vi "Set Message2 Text Html.vi"(0 "handles cluster in":T1 caption="ハンドルクラスター入力", 5 "subject":string caption="件名", 7 "plain text message":string caption="標準テキストメッセージ", 9 "html message":string caption="htmlメッセージ", 11 "error in (no error)":errorcluster caption="エラー入力（エラーなし）") -> (4 "handles cluster out":T1 caption="ハンドルクラスター出力", 15 "error out":errorcluster caption="エラー出力")   [LabVIEW 2015]
doc: "Eメールの本文に含めるテキストとHTMLを設定します。\nメールは「multipart」となり、標準テキストメッセージが「content-type: text/plain」に、htmlメッセージが「content-type: text/html」となる。"
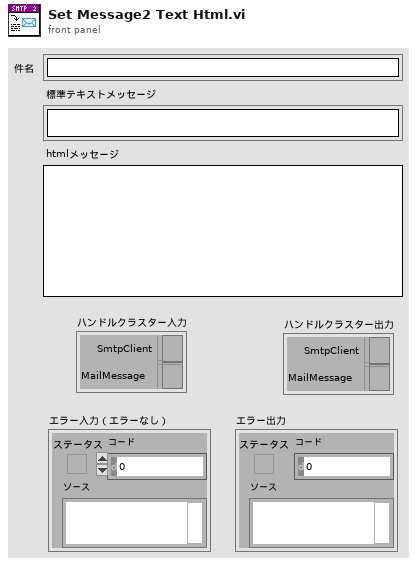
[diagram p1: front panel]
types:
  T1 = cluster{"SmtpClient":refnum<k24>, "MailMessage":refnum<k24>}
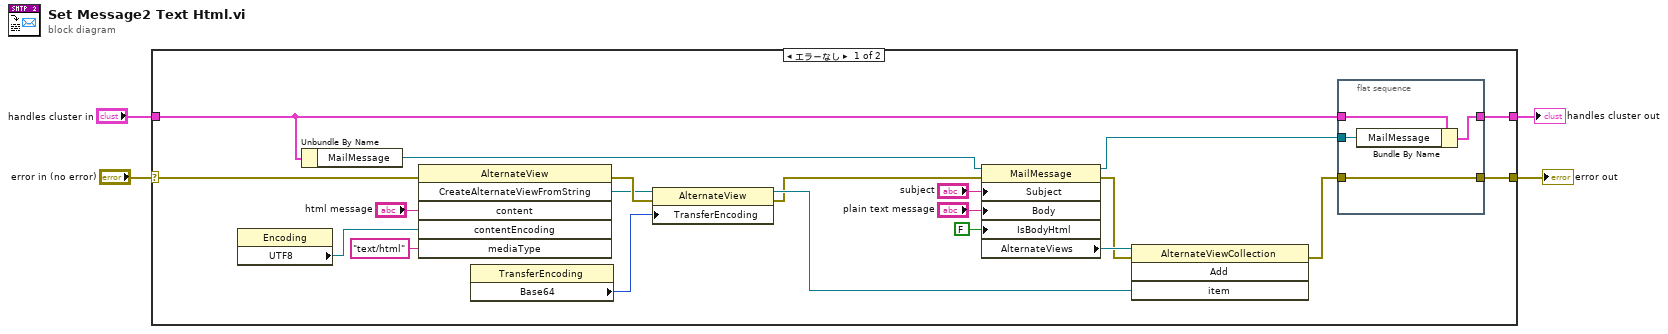
[diagram p0: block diagram]
diagram:
  n1 = case shown="エラーなし" "error in (no error)" {
    selector: "error in (no error)" -> [w16 w30]
    tunnel: [w12 w30] -> w3
    tunnel: "handles cluster in" -> [w24 w29]
    tunnel: [w23 w29] -> w1
    frame No Error {
      n2 = property class="Encoding"() -> ("UTF8"=w10:refnum<k24>)  [unwired: 2 in, 2 out]
      n3 = Unbundle By Name(w24) -> ("MailMessage"=w22:refnum<k24>)
      n4 = invoke class="AlternateView" method="CreateAlternateViewFromString"(error in=w16, "content"="html message", "contentEncoding"=w10, "mediaType"="text/html") -> (error out=w9:errorcluster, "CreateAlternateViewFromString"=w8:refnum<k24>)  [unwired: 2 in, 4 out]
      n5 = property class="TransferEncoding"() -> ("Base64"=w7:i32)  [unwired: 2 in, 2 out]
      n6 = property class="AlternateView"(reference=w8, error in=w9, "TransferEncoding"=w7) -> (reference out=w6:refnum<k24>, error out=w5:errorcluster)
      n7 = property class="MailMessage"(reference=w22, error in=w5, "Subject"="subject", "Body"="plain text message", "IsBodyHtml"=FALSE) -> (reference out=w20:refnum<k24>, error out=w14:errorcluster, "AlternateViews"=w15:refnum<k24>)
      n8 = invoke class="AlternateViewCollection" method="Add"(reference=w15, error in=w14, "item"=w6) -> (error out=w13:errorcluster)  [unwired: 1 in, 3 out]
      n9 = flat-sequence {
        tunnel: w24 -> [w28]
        tunnel: [w27] -> w23
        tunnel: w20 -> [w26]
        tunnel: w13 -> [w25]
        tunnel: [w25] -> w12
        frame #0 {
          n10 = Bundle By Name(cluster=w28, "MailMessage"=w26) -> (w27:T1)
        }
      }
    }
    frame Error {
    }
  }
  "handles cluster out" <- w1
  "error out" <- w3
